vi "MouseClick.vi"(0 "VI Reference In":refnum<vi>, 7 "Control Path":string, 11 "error In":errorcluster) -> (4 "VI Reference Out":refnum<vi>, 15 "error out":errorcluster)   [LabVIEW 2016]
uses:
  main/apis/Setup/GetControlRef/GetControlRefByPath.vi
  main/apis/Setup/GetControlRef/GetControlRef.lvlib
  User32.dll
  main/Drona.lvlib
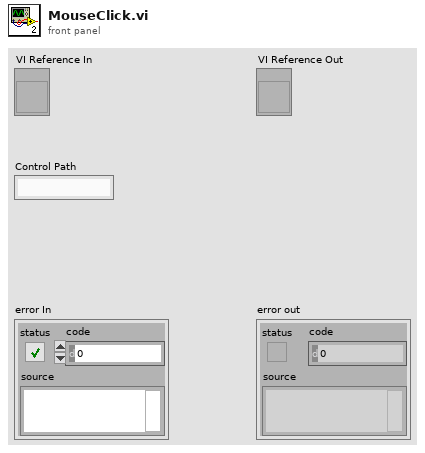
[diagram p1: front panel]
types:
  T1 = typedef "LVPositionTypeDef.ctl" = cluster{"Left":i32, "Top":i32}
  T2 = typedef "LVRectTypeDef.ctl" = cluster{"Left":i16, "Top":i16, "Right":i16, "Bottom":i16}
  T3 = typedef "LVPointTypeDef.ctl" = cluster{"Horizontal":i16, "Vertical":i16}
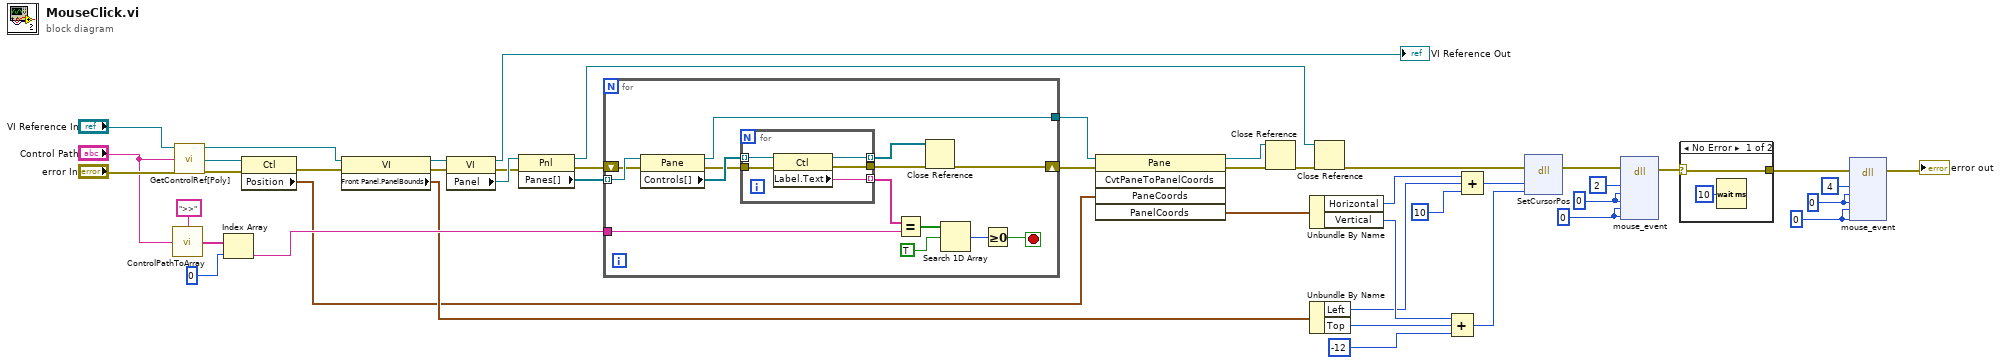
[diagram p0: block diagram]
diagram:
  w9 = 0 ("dwExtraInfo")
  w10 = u32 0 ("dwExtraInfo")
  w8 = 0 ("dwExtraInfo")
  w7 = u32 0 ("dwExtraInfo")
  n1 = call "ControlPathToArray.vi"("Control Name"="Control Path", "delimiter (>>)"=">>") -> ("Control Path"=w26:string[])
  n2 = call-poly "GetControlRef[Poly].vi"("VI Reference In"="VI Reference In", "Control Path"="Control Path", "error In"="error In") -> ("VI Reference Out"=w13:refnum<vi>, "Ctl Refnum"=w38:refnum<vi>, "error out"=w40:errorcluster)  [unwired: 10 in]
  n3 = Index Array(array=w26, index=0) -> (element=w24:string)
  n4 = property class="Ctl"(reference=w38, error in=w40) -> (error out=w21:errorcluster, "Position"=w14:T1)  [unwired: 1 out]
  n5 = property class="VI"(reference=w13, error in=w21) -> (reference out=w22:refnum<vi>, error out=w20:errorcluster, "Front Panel.PanelBounds"=w19:T2)
  n6 = property class="VI"(reference=w22, error in=w20) -> (reference out=→"VI Reference Out":refnum<vi>, error out=w44:errorcluster, "Panel"=w45:refnum<vi>)
  n7 = property class="Pnl"(reference=w45, error in=w44) -> (reference out=w36:refnum<vi>, error out=w42:errorcluster, "Panes[]"=w43:refnum<vi>[])
  n8 = for {
    tunnel: w43 -> [w60] mode=indexing
    tunnel: [w51] -> w32
    shift-right: [w48] -> w41
    shift-left: w42 -> [w59]
    tunnel: w24 -> [w56]
    stop <- w52 stop-if-true
    n9 = property class="Pane"(reference=w60, error in=w59) -> (reference out=w51:refnum<vi>, error out=w50:errorcluster, "Controls[]"=w58:refnum<vi>[])
    n10 = for {
      tunnel: w58 -> [w65] mode=indexing
      tunnel: [w64] -> w57 mode=indexing
      tunnel: w50 -> [w63]
      tunnel: [w62] -> w49
      tunnel: [w61] -> w47 mode=indexing
      n11 = property class="Ctl"(reference=w65, error in=w63) -> (reference out=w61:refnum<vi>, error out=w62:errorcluster, "Label.Text"=w64:string)
    }
    n12 = Equal?(x=w57, y=w56) -> (x = y?=w55:bool[])
    n13 = Close Reference(reference=w47, error in (no error)=w49) -> (error out=w48:errorcluster)
    n14 = Search 1D Array(1D array=w55, element=TRUE) -> (index of element=w53:i32)  [unwired: 1 in]
    n15 = Greater Or Equal To 0?(x=w53) -> (x >= 0?=w52:bool)
  }
  n16 = invoke class="Pane" method="CvtPaneToPanelCoords"(reference=w32, error in=w41, "PaneCoords"=w14) -> (reference out=w33:refnum<vi>, error out=w46:errorcluster, "PanelCoords"=w35:T3)  [unwired: 2 in, 2 out]
  n17 = Close Reference(reference=w33, error in (no error)=w46) -> (error out=w37:errorcluster)
  n18 = Unbundle By Name(w35) -> ("Horizontal"=w31:i16, "Vertical"=w29:i16)
  n19 = Unbundle By Name(w19) -> ("Left"=w17:i16, "Top"=w18:i16)
  n20 = Close Reference(reference=w36, error in (no error)=w37) -> (error out=w2:errorcluster)
  n21 = Compound Arithmetic op=ADD(w29, w18, i16 -12 ("value")) -> (w28:i16)
  n22 = Compound Arithmetic op=ADD(w31, w17, i16 10 ("value")) -> (w30:i16)
  n23 = dll-call lib="user32.dll" fn="SetCursorPos" label="Move mouse"(error in=w2, "dx"=w30, "dy"=w28) -> (error out=w3:errorcluster)  [unwired: 5 in, 1 out]
  n24 = dll-call lib="user32.dll" fn="mouse_event" label="Click"(error in=w3, "dwFlags"=2, "dx"=w8, "dy"=w8, "dwData"=w7, "dwExtraInfo"=w7) -> (error out=w5:errorcluster)  [unwired: 8 in, 1 out]
  n25 = case shown="No Error" w5 {
    selector: w5 -> [w66 w68]
    tunnel: [w66 w68] -> w4
    frame No Error {
      n26 = Wait (ms)(milliseconds to wait=u32 10) -> ()  [unwired: 1 out]
    }
    frame Error {
    }
  }
  n27 = dll-call lib="user32.dll" fn="mouse_event" label="Release"(error in=w4, "dwFlags"=4, "dx"=w9, "dy"=w9, "dwData"=w10, "dwExtraInfo"=w10) -> (error out=→"error out":errorcluster)  [unwired: 8 in, 1 out]
